vi "Service.Create.vi"(7 "Type":T1, 8 "error in (no error)":errorcluster, 10 "Variant":variant, 11 "Section Ptr":T2 format="%.0x") -> (0 "error out":errorcluster, 3 "Parent Ref out":T2 format="%.0x")   [LabVIEW 2019, in "Diagnostics Addon System Explorer.lvlib"]
uses:
  Diagnostics Addon System Explorer.lvlib
  <vilib>/NI VeriStand/Custom Device API/Custom Device Item Ref.ctl
  Addon Shared/Types/Type.ctl
  Types/Frame.Export.ctl
  Addon Shared/Types/Signal.ctl
  Types/FG.Action.ctl
  Types/CmdResp.Export.ctl
  Types/IO.Export.ctl
  Types/Poll.Create.ctl
  Types/Poll.Settings.ctl
  Types/Poll.LinkedNode.ctl
  Addon Shared/Types/DPID.Rate.ctl
  Addon Shared/Types/DPID.ctl
  Types/UserDefinedMessage.Export.ctl
  Addon Shared/Types/Security.ctl
  Addon Shared/Types/Security.Type.ctl
  <vilib>/NI VeriStand/Custom Device API/Custom Device Channel.ctl
  <vilib>/NI VeriStand/Custom Device API/Custom Device Channel Type.ctl
  Addon Shared/Types/DTC.Settings.ctl
  Addon Shared/Types/DTC.Descriptor.ctl
  FileDependency.Create.vi
  Addon Shared/SubVIs/Constants.vi
  <vilib>/NI/NI VeriStand Advanced SysDef API/SysDef API/SysDef.Property.Set.vi
  <vilib>/NI/NI VeriStand Advanced SysDef API/_SubVIs/SysDef.Property.Set.U32.vi
  <vilib>/NI VeriStand/Custom Device API/NI VeriStand - Get Item Property.vi
  <vilib>/NI VeriStand/Custom Device API/Get Item Property (U32).vi
  <vilib>/NI/NI VeriStand Advanced SysDef API/_SubVIs/SysDef.Property.Set.U32.Array.vi
  <vilib>/NI VeriStand/Custom Device API/Get Item Property (U32 Array).vi
  FileDependency.Get.Target Path.vi
  <vilib>/Utility/MD5Checksum.llb/MD5Checksum File.vi
  <vilib>/NI/NI VeriStand Advanced SysDef API/_SubVIs/SysDef.Property.Set.DependentFile.vi
  <vilib>/NI/NI VeriStand Advanced SysDef API/SysDef API/SysDef.Property.Remove.vi
  <vilib>/NI/NI VeriStand Advanced SysDef API/_SubVIs/SysDef.Property.Set.I32.vi
  <vilib>/NI/NI VeriStand Advanced SysDef API/_SubVIs/SysDef.Property.Set.DBL.Array.vi
  <vilib>/NI/NI VeriStand Advanced SysDef API/_SubVIs/SysDef.Property.Set.String.Array.vi
  <vilib>/NI VeriStand/Custom Device API/Get Item Property (I32).vi
  <vilib>/NI VeriStand/Custom Device API/Get Item Property (Double Array).vi
  <vilib>/NI VeriStand/Custom Device API/Get Item Property (String Array).vi
  Addon Shared/Diagnostics Addon Shared.lvlib
  <vilib>/NI/NI VeriStand Advanced SysDef API/SysDef API/Advanced System Definition.lvlib
  <vilib>/NI VeriStand/Custom Device API/Custom Device API.lvlib
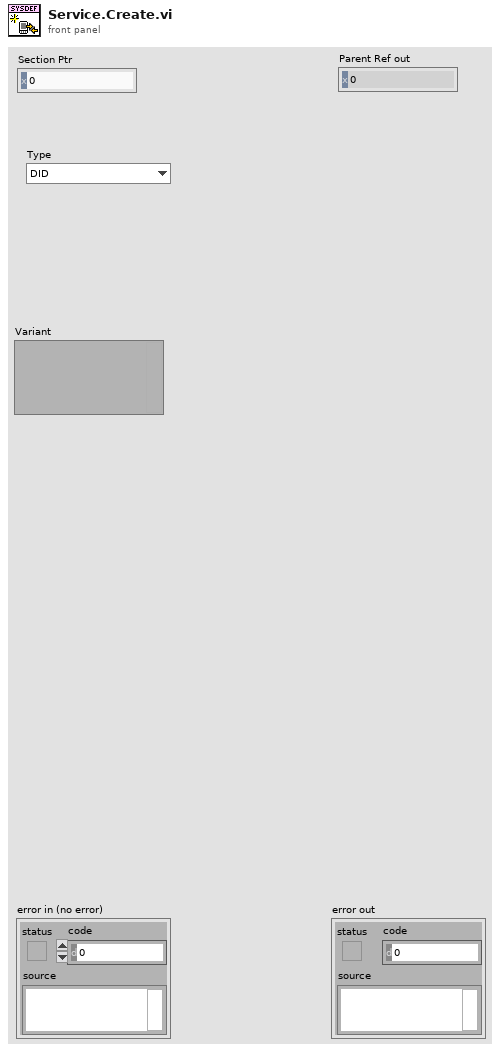
[diagram p1: front panel]
types:
  T1 = typedef "Diagnostics Addon Shared.lvlib/Type.ctl" = enum16{"DID", "CDID", "PID", "CPID", "Read Memory", "Write Memory", "IO Control", "Routine Start", "Routine Request", "Routine Stop", "User Defined", "DTC Control", "Clear DTCs", "Read DTCs", "Start DTCs", "DTC Change Count", "Tester Present", "Unlock ECU", "Reset ECU", "Diag Session Control", "Communication Control", "DPID Control", "Poll Control", "Diag CAN Control"}
  T2 = typedef "Custom Device API.lvlib/Custom Device Item Ref.ctl" = u64
  T3 = typedef "Diagnostics Addon System Explorer.lvlib/Frame.Export.ctl" = cluster{"Name":string, "ID":u32, "Signals":T4[]}
  T4 = typedef "Diagnostics Addon Shared.lvlib/Signal.ctl" = cluster{"Start Bit":u32, "Length":u32, "Scaling Factor":dbl, "Scaling Offset":dbl, "Minimum":dbl, "Maximum":dbl, "Data Type":u32, "Byte Order":u32, "Default Value":dbl, "Name":string, "Units":string}
  T5 = typedef "Diagnostics Addon System Explorer.lvlib/FG.Action.ctl" = enum16{"Get", "Set"}
  T6 = typedef "Diagnostics Addon System Explorer.lvlib/CmdResp.Export.ctl" = cluster{"Cmd":T4[], "Response":T4[]}
  T7 = typedef "Diagnostics Addon System Explorer.lvlib/IO.Export.ctl" = cluster{"Name":string, "ID":u16, "Signals":T6}
  T8 = typedef "Diagnostics Addon System Explorer.lvlib/Poll.Create.ctl" = cluster{"Name":string, "Settings":T9}
  T9 = typedef "Diagnostics Addon System Explorer.lvlib/Poll.Settings.ctl" = cluster{"Input Channels":T10[], "Speed":T11}
  T10 = typedef "Diagnostics Addon System Explorer.lvlib/Poll.LinkedNode.ctl" = cluster{"Node ID":u64}
  T11 = typedef "Diagnostics Addon Shared.lvlib/DPID.Rate.ctl" = enum16{"Slow", "Medium", "Fast"}
  T12 = typedef "Diagnostics Addon Shared.lvlib/DPID.ctl" = cluster{"DPID ID":u8, "Speed":T11, "PIDs":u16[]}
  T13 = typedef "Diagnostics Addon System Explorer.lvlib/UserDefinedMessage.Export.ctl" = cluster{"Name":string, "Signals":T6}
  T14 = typedef "Diagnostics Addon Shared.lvlib/Security.ctl" = cluster{"Type":T15, "Source DLL Path":path, "Target DLL Path":path, "Security Level":u8}
  T15 = typedef "Diagnostics Addon Shared.lvlib/Security.Type.ctl" = enum16{"None", "DLL", "MasterKey"}
  T16 = typedef "Custom Device API.lvlib/Custom Device Channel.ctl" = cluster{"Type":T17, "Units":string, "Default Value":dbl, "Faultable":bool, "Scalable":bool}
  T17 = typedef "Custom Device API.lvlib/Custom Device Channel Type.ctl" = enum16{"Input", "Output"}
  T18 = typedef "Diagnostics Addon Shared.lvlib/DTC.Settings.ctl" = cluster{"Descriptor":T19, "Value.Code":dbl[], "Value.String":string[], "Value.J2012String":string[], "Status.Code":dbl[], "Status.String":string[]}
  T19 = typedef "Diagnostics Addon Shared.lvlib/DTC.Descriptor.ctl" = cluster{"DTC Byte Length":i32, "Status Byte Length":i32, "Add Data Byte Length":i32, "Byte Order":enum16{"Motorola", "Intel"}}
  T20 = typedef "Diagnostics Addon Shared.lvlib/Protocol.ctl" = enum16{"GMLAN", "KWP-2000", "UDS", "User-Defined"}
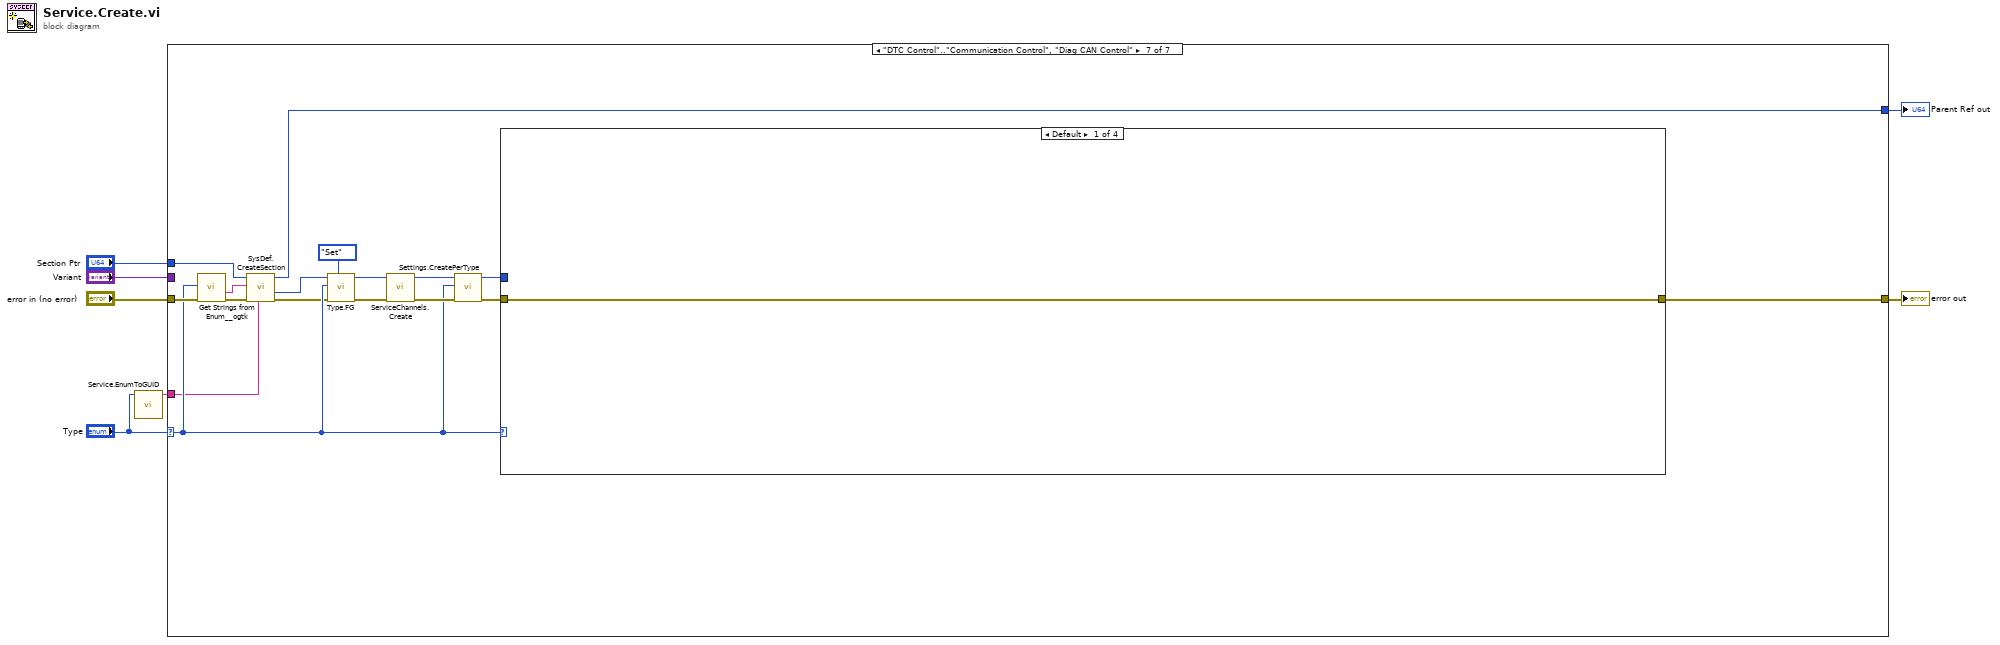
[diagram p0: block diagram]
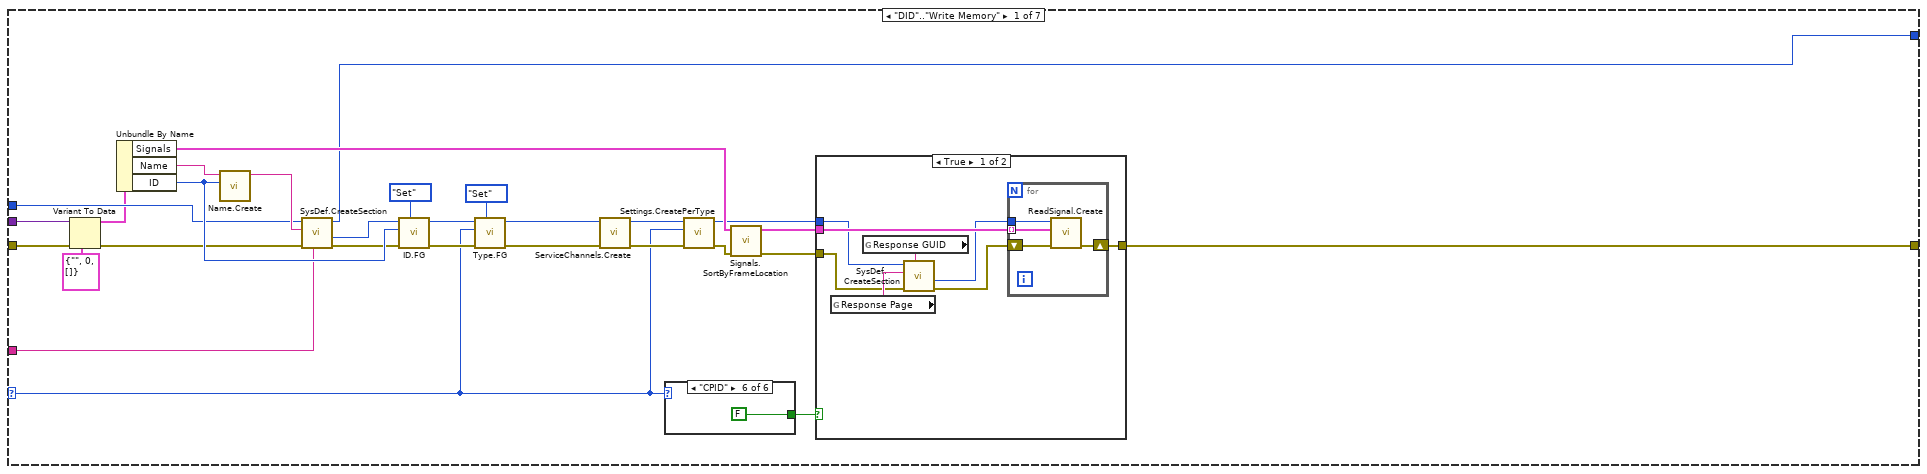
[diagram p2: hidden frame]
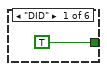
[diagram p3: hidden frame]
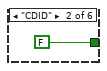
[diagram p4: hidden frame]
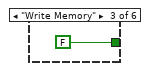
[diagram p5: hidden frame]
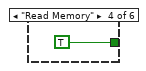
[diagram p6: hidden frame]
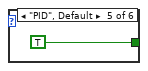
[diagram p7: hidden frame]
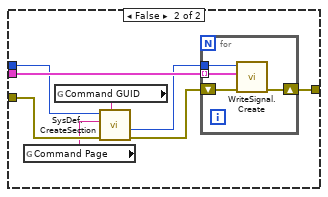
[diagram p8: hidden frame]
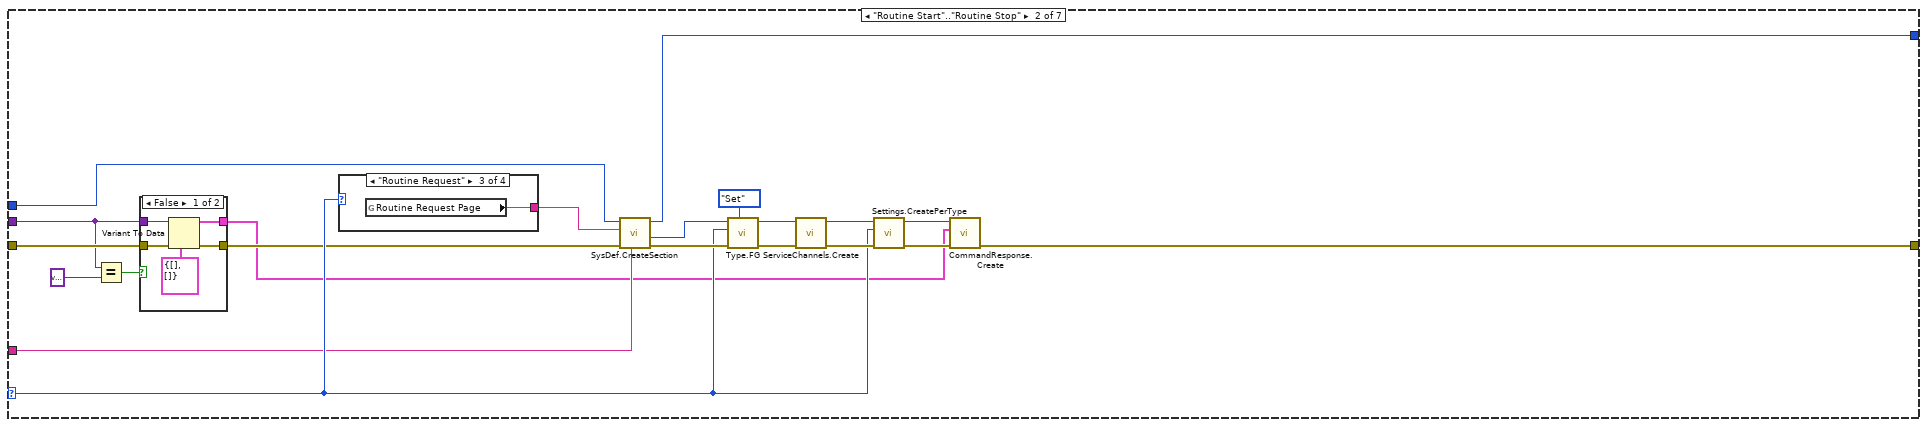
[diagram p9: hidden frame]
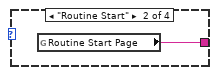
[diagram p12: hidden frame]
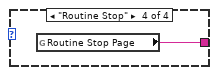
[diagram p13: hidden frame]
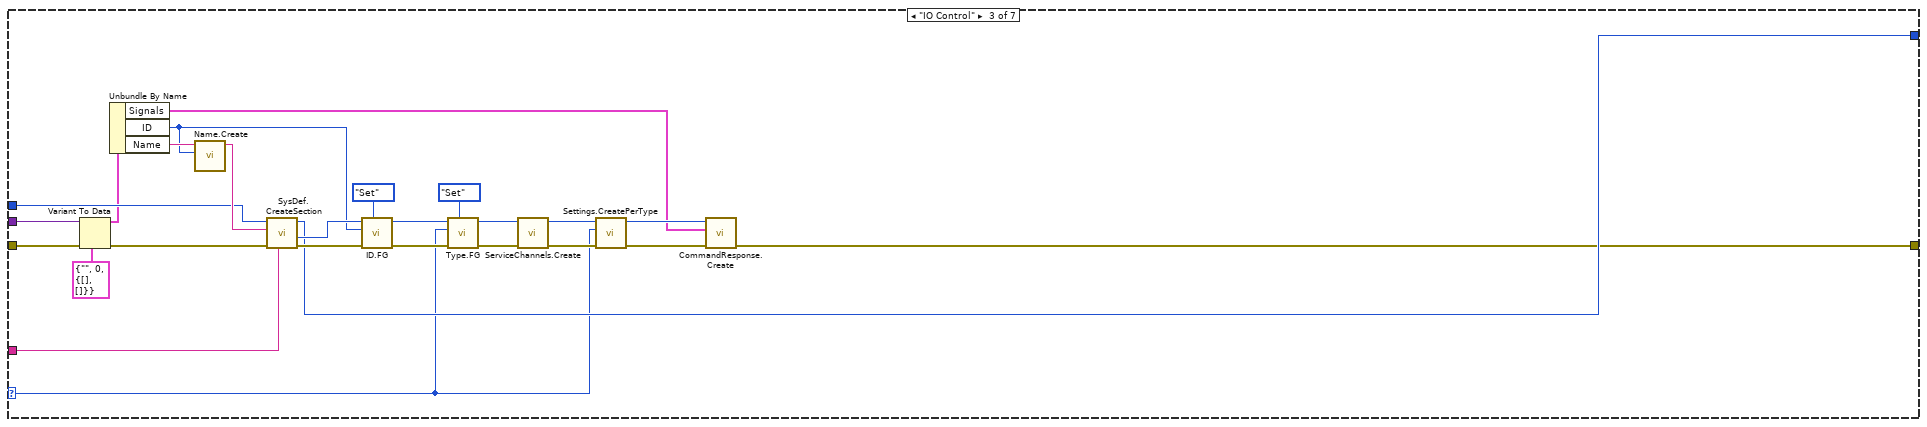
[diagram p14: hidden frame]
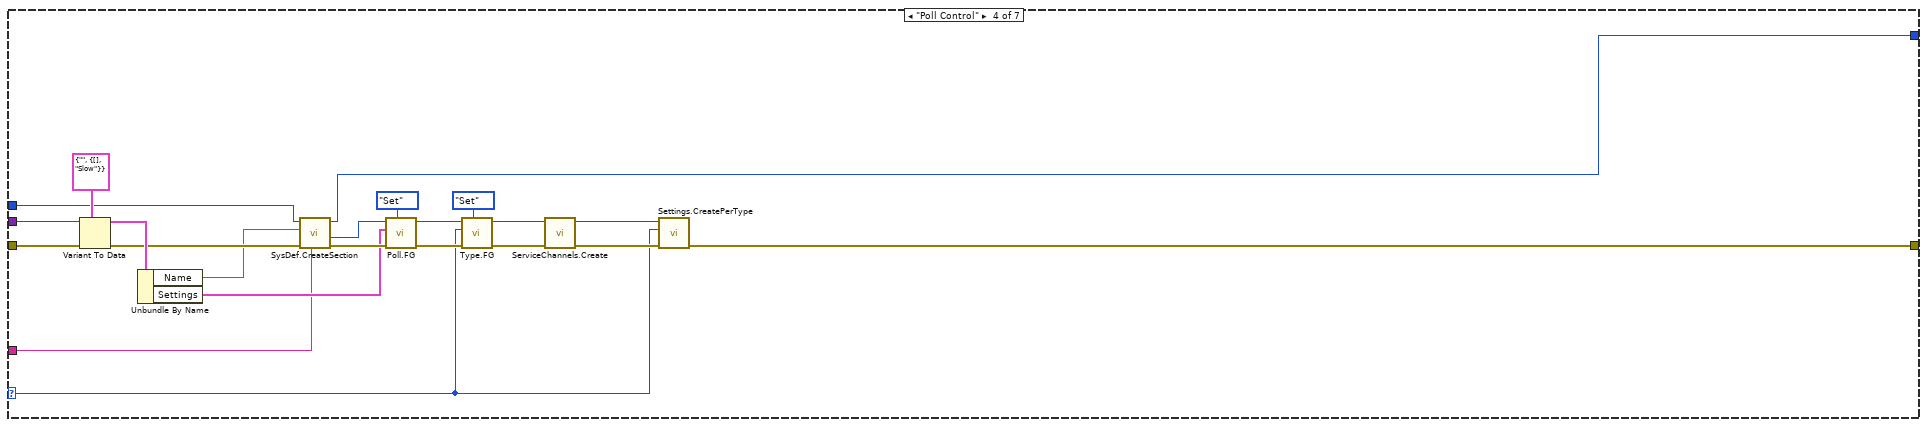
[diagram p15: hidden frame]
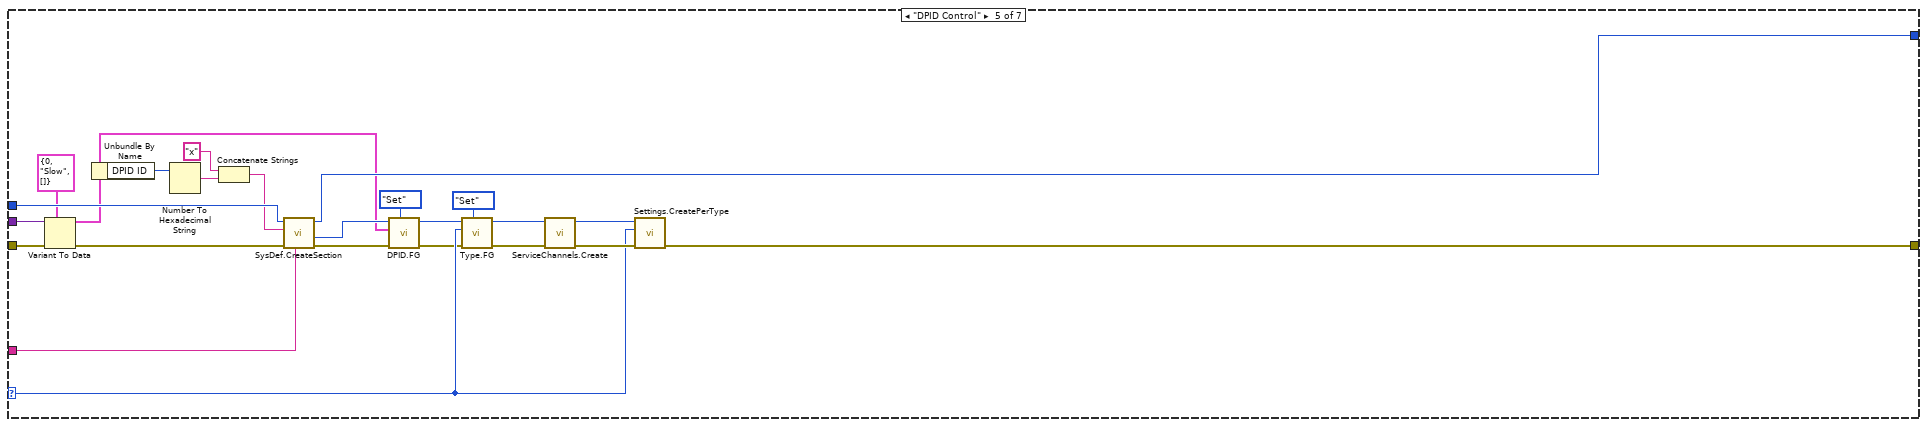
[diagram p16: hidden frame]
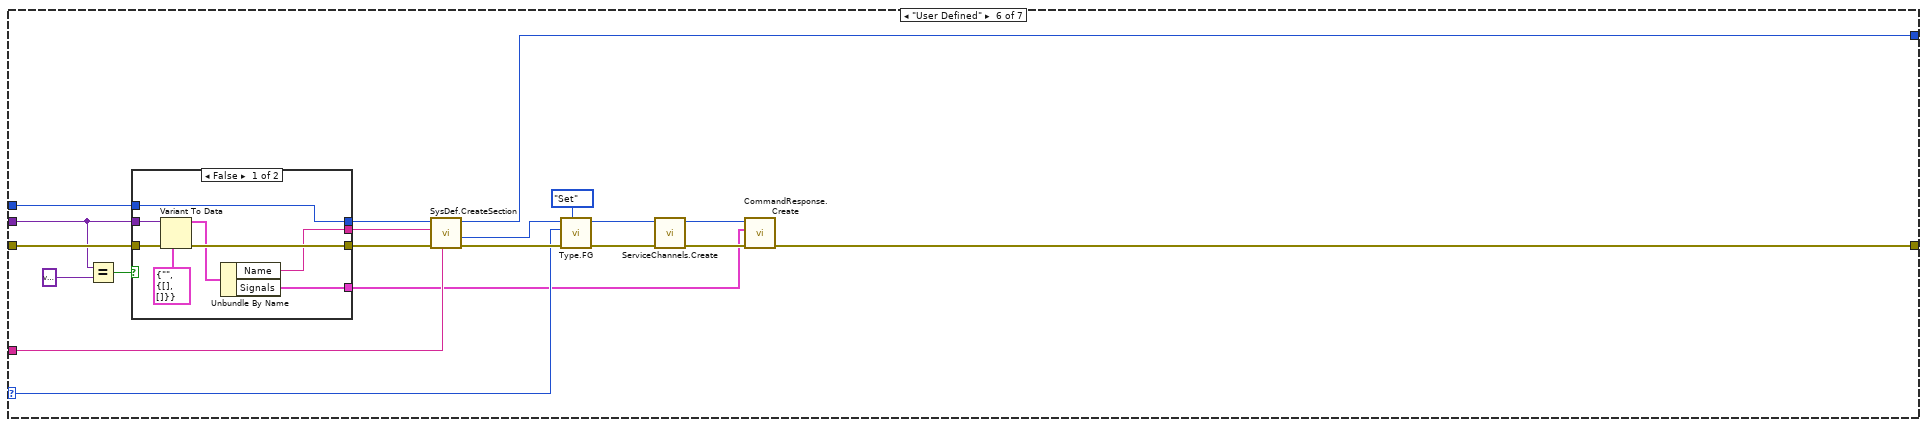
[diagram p17: hidden frame]
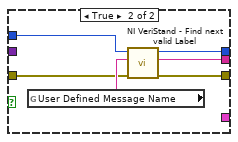
[diagram p18: hidden frame]
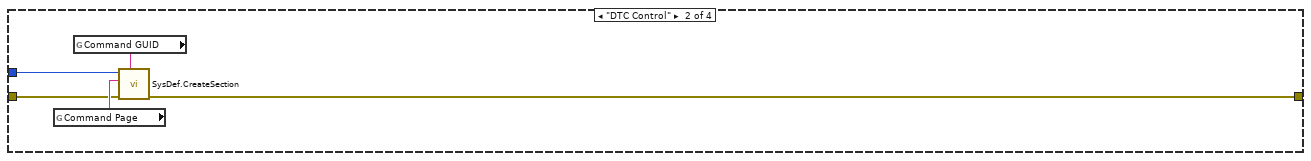
[diagram p19: hidden frame]
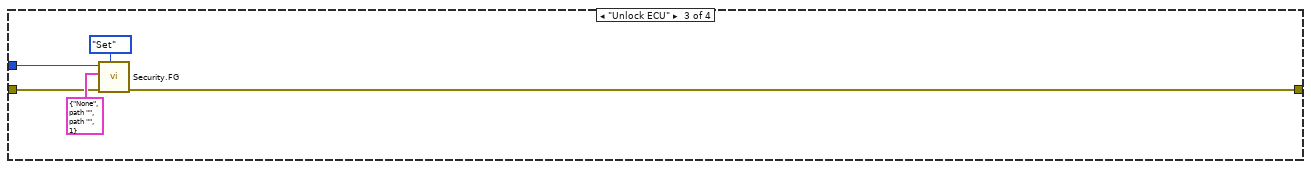
[diagram p20: hidden frame]
diagram:
  n1 = call "Service.EnumToGUID.vi"("Type"="Type") -> ("GUID"=w1:string)  [unwired: 10 in]
  n2 = case shown="\"DTC Control\"..\"Communication Control\", \"Diag CAN Control\"" "Type" {
    selector: "Type" -> [w17 w75 w101 w123 w156 w179 w212]
    tunnel: "error in (no error)" -> [w19 w72 w112 w144 w168 w175 w215]
    tunnel: "Section Ptr" -> [w18 w67 w116 w136 w165 w172 w208]
    tunnel: [w16 w87 w114 w124 w157 w188 w211] -> w5
    tunnel: [w15 w85 w115 w135 w164 w187 w210] -> w4
    tunnel: "Variant" -> [w13 w70 w111 w143 w167 w174 _]
    tunnel: w1 -> [w10 w74 w98 w132 w163 w178 w203]
    frame "DID".."Write Memory" {
      n3 = Variant To Data(error in=w19, type=T3 {"Name"="", "ID"=0, "Signals"=[]} ("Frame"), Variant=w13) -> (data=w11:T3, error out=w14:errorcluster)
      n4 = Unbundle By Name(w11) -> ("Signals"=w25:T4[], "Name"=w32:string, "ID"=w34:u32)
      n5 = call "Name.Create.vi"("PID Number"=w34, "PID Name"=w32) -> ("VS Name"=w36:string)  [unwired: 9 in]
      n6 = call <vilib>:"SysDef.CreateSection.vi"("GUID"=w10, "error in (no error)"=w14, "Name"=w36, "nodeID"=w18) -> ("error out"=w29:errorcluster, "New NodeID"=w30:u64, "nodeID out"=w15:u64)  [unwired: 4 in, 1 out]
      n7 = call "ID.FG.vi"("Action"=FG.Action."Set", "error in (no error)"=w29, "ID"=w34, "Device Item Ref in"=w30) -> ("error out"=w28:errorcluster, "Device Item Ref out"=w27:T2)  [unwired: 5 in, 1 out]
      n8 = call "Type.FG.vi"("Action"=FG.Action."Set", "error in (no error)"=w28, "Type"=w17, "Device Item Ref in"=w27) -> ("error out"=w9:errorcluster, "Device Item Ref out"=w8:T2)  [unwired: 5 in, 1 out]
      n9 = call "ServiceChannels.Create.vi"("error in (no error)"=w9, "nodeID in"=w8) -> ("error out"=w20:errorcluster, "nodeID out"=w22:u64)  [unwired: 8 in]
      n10 = case shown="\"CPID\"" w17 {
        tunnel: [TRUE FALSE FALSE TRUE TRUE FALSE] -> w31
        frame "DID" {
        }
        frame "CDID" {
        }
        frame "Write Memory" {
        }
        frame "Read Memory" {
        }
        frame "PID", Default {
        }
        frame "CPID" {
        }
      }
      n11 = call "Settings.CreatePerType.vi"("error in (no error)"=w20, "Type"=w17, "nodeID in"=w22) -> ("error out"=w21:errorcluster, "nodeID out"=w23:u64)  [unwired: 7 in]
      n12 = call "Signals.SortByFrameLocation.vi"("error in (no error)"=w21, "Signals in"=w25) -> ("error out"=w26:errorcluster, "Signals out"=w24:T4[])  [unwired: 8 in]
      n13 = case shown="True" w31 {
        tunnel: w23 -> [w43 w59]
        tunnel: w24 -> [w50 w62]
        tunnel: [w49 w61] -> w16
        tunnel: w26 -> [w45 w60]
        frame True {
          n14 = global read "Constants.vi" "Response Page"() -> (w47:string)
          n15 = global read "Constants.vi" "Response GUID"() -> (w48:string)
          n16 = call <vilib>:"SysDef.CreateSection.vi"("GUID"=w48, "error in (no error)"=w45, "Name"=w47, "nodeID"=w43) -> ("error out"=w46:errorcluster, "New NodeID"=w44:u64)  [unwired: 4 in, 2 out]
          n17 = for {
            shift-right: [w53] -> w49
            shift-left: w46 -> [w54]
            tunnel: w50 -> [w51] mode=indexing
            tunnel: w44 -> [w52]
            n18 = call "ReadSignal.Create.vi"("error in (no error)"=w54, "Signal Parameters"=w51, "Section Ptr"=w52) -> ("error out"=w53:errorcluster)  [unwired: 7 in, 1 out]
          }
        }
        frame False {
          n19 = global read "Constants.vi" "Command Page"() -> (w55:string)
          n20 = global read "Constants.vi" "Command GUID"() -> (w56:string)
          n21 = call <vilib>:"SysDef.CreateSection.vi"("GUID"=w56, "error in (no error)"=w60, "Name"=w55, "nodeID"=w59) -> ("error out"=w57:errorcluster, "New NodeID"=w58:u64)  [unwired: 4 in, 2 out]
          n22 = for {
            shift-right: [w63] -> w61
            shift-left: w57 -> [w65]
            tunnel: w62 -> [w64] mode=indexing
            tunnel: w58 -> [w66]
            n23 = call "WriteSignal.Create.vi"("error in (no error)"=w65, "Signal Parameters"=w64, "Section Ptr"=w66) -> ("error out"=w63:errorcluster)  [unwired: 7 in, 1 out]
          }
        }
      }
    }
    frame "Routine Start".."Routine Stop" {
      n24 = Equal?(x=w70, y=variant) -> (x = y?=w68:bool)
      n25 = case shown="False" w68 {
        tunnel: [w92 w93] -> w73
        tunnel: w72 -> [w91 w93]
        tunnel: [w89 _] -> w71
        tunnel: w70 -> [w88 _]
        frame False {
          n26 = Variant To Data(error in=w91, type=T6 {"Cmd"=[], "Response"=[]} ("Start Parameters"), Variant=w88) -> (data=w89:T6, error out=w92:errorcluster)
        }
        frame True {
        }
      }
      n27 = case shown="\"Routine Request\"" w75 {
        tunnel: [_ w94 w95 w96] -> w86
        frame Default {
        }
        frame "Routine Start" {
          n28 = global read "Constants.vi" "Routine Start Page"() -> (w94:string)
        }
        frame "Routine Request" {
          n29 = global read "Constants.vi" "Routine Request Page"() -> (w95:string)
        }
        frame "Routine Stop" {
          n30 = global read "Constants.vi" "Routine Stop Page"() -> (w96:string)
        }
      }
      n31 = call <vilib>:"SysDef.CreateSection.vi"("GUID"=w74, "error in (no error)"=w73, "Name"=w86, "nodeID"=w67) -> ("error out"=w78:errorcluster, "New NodeID"=w79:u64, "nodeID out"=w85:u64)  [unwired: 4 in, 1 out]
      n32 = call "Type.FG.vi"("Action"=FG.Action."Set", "error in (no error)"=w78, "Type"=w75, "Device Item Ref in"=w79) -> ("error out"=w77:errorcluster, "Device Item Ref out"=w76:T2)  [unwired: 5 in, 1 out]
      n33 = call "ServiceChannels.Create.vi"("error in (no error)"=w77, "nodeID in"=w76) -> ("error out"=w84:errorcluster, "nodeID out"=w83:u64)  [unwired: 8 in]
      n34 = call "Settings.CreatePerType.vi"("error in (no error)"=w84, "Type"=w75, "nodeID in"=w83) -> ("error out"=w81:errorcluster, "nodeID out"=w80:u64)  [unwired: 7 in]
      n35 = call "CommandResponse.Create.vi"("error in (no error)"=w81, "Signals"=w71, "New NodeID"=w80) -> ("error out"=w87:errorcluster)  [unwired: 8 in]
    }
    frame "IO Control" {
      n36 = Variant To Data(error in=w112, type=T7 {"Name"="", "ID"=0, "Signals"={"Cmd"=[], "Response"=[]}} ("IO Control"), Variant=w111) -> (data=w110:T7, error out=w113:errorcluster)
      n37 = Unbundle By Name(w110) -> ("Signals"=w97:T6, "ID"=w118:u16, "Name"=w121:string)
      n38 = call "Name.Create.vi"("PID Number"=w118, "PID Name"=w121) -> ("VS Name"=w122:string)  [unwired: 9 in]
      n39 = call <vilib>:"SysDef.CreateSection.vi"("GUID"=w98, "error in (no error)"=w113, "Name"=w122, "nodeID"=w116) -> ("error out"=w120:errorcluster, "New NodeID"=w119:u64, "nodeID out"=w115:u64)  [unwired: 4 in, 1 out]
      n40 = call "ID.FG.vi"("Action"=FG.Action."Set", "error in (no error)"=w120, "ID"=w118, "Device Item Ref in"=w119) -> ("error out"=w103:errorcluster, "Device Item Ref out"=w100:T2)  [unwired: 5 in, 1 out]
      n41 = call "Type.FG.vi"("Action"=FG.Action."Set", "error in (no error)"=w103, "Type"=w101, "Device Item Ref in"=w100) -> ("error out"=w102:errorcluster, "Device Item Ref out"=w99:T2)  [unwired: 5 in, 1 out]
      n42 = call "ServiceChannels.Create.vi"("error in (no error)"=w102, "nodeID in"=w99) -> ("error out"=w108:errorcluster, "nodeID out"=w107:u64)  [unwired: 8 in]
      n43 = call "Settings.CreatePerType.vi"("error in (no error)"=w108, "Type"=w101, "nodeID in"=w107) -> ("error out"=w105:errorcluster, "nodeID out"=w106:u64)  [unwired: 7 in]
      n44 = call "CommandResponse.Create.vi"("error in (no error)"=w105, "Signals"=w97, "New NodeID"=w106) -> ("error out"=w114:errorcluster)  [unwired: 8 in]
    }
    frame "Poll Control" {
      n45 = Variant To Data(error in=w144, type=T8 {"Name"="", "Settings"={"Input Channels"=[], "Speed"=enum."Slow"}} ("output cluster"), Variant=w143) -> (data=w141:T8, error out=w137:errorcluster)
      n46 = Unbundle By Name(w141) -> ("Name"=w134:string, "Settings"=w133:T9)
      n47 = call <vilib>:"SysDef.CreateSection.vi"("GUID"=w132, "error in (no error)"=w137, "Name"=w134, "nodeID"=w136) -> ("error out"=w139:errorcluster, "New NodeID"=w138:u64, "nodeID out"=w135:u64)  [unwired: 4 in, 1 out]
      n48 = call "Poll.FG.vi"("Action"=FG.Action."Set", "error in"=w139, "Selected Channels"=w133, "Parent Ref"=w138) -> ("error out"=w130:errorcluster, "Parent Ref Out"=w128:T2)  [unwired: 5 in, 1 out]
      n49 = call "Type.FG.vi"("Action"=FG.Action."Set", "error in (no error)"=w130, "Type"=w123, "Device Item Ref in"=w128) -> ("error out"=w129:errorcluster, "Device Item Ref out"=w127:T2)  [unwired: 5 in, 1 out]
      n50 = call "ServiceChannels.Create.vi"("error in (no error)"=w129, "nodeID in"=w127) -> ("error out"=w126:errorcluster, "nodeID out"=w125:u64)  [unwired: 8 in]
      n51 = call "Settings.CreatePerType.vi"("error in (no error)"=w126, "Type"=w123, "nodeID in"=w125) -> ("error out"=w124:errorcluster)  [unwired: 7 in, 1 out]
    }
    frame "DPID Control" {
      n52 = Variant To Data(error in=w168, type=T12 {"DPID ID"=0, "Speed"=enum."Slow", "PIDs"=[]} ("DPID"), Variant=w167) -> (data=w145:T12, error out=w166:errorcluster)
      n53 = Unbundle By Name(w145) -> ("DPID ID"=w153:u8)
      n54 = Number To Hexadecimal String(2:w153) -> (0:w155:string)  [unwired: 1 in]
      n55 = Concatenate Strings("x" ("string"), w155) -> (w151:string)
      n56 = call <vilib>:"SysDef.CreateSection.vi"("GUID"=w163, "error in (no error)"=w166, "Name"=w151, "nodeID"=w165) -> ("error out"=w149:errorcluster, "New NodeID"=w148:u64, "nodeID out"=w164:u64)  [unwired: 4 in, 1 out]
      n57 = call "DPID.FG.vi"("Action"=FG.Action."Set", "error in (no error)"=w149, "DPID"=w145, "Device Item Ref in"=w148) -> ("error out"=w150:errorcluster, "Device Item Ref out"=w147:T2)  [unwired: 5 in, 1 out]
      n58 = call "Type.FG.vi"("Action"=FG.Action."Set", "error in (no error)"=w150, "Type"=w156, "Device Item Ref in"=w147) -> ("error out"=w161:errorcluster, "Device Item Ref out"=w160:T2)  [unwired: 5 in, 1 out]
      n59 = call "ServiceChannels.Create.vi"("error in (no error)"=w161, "nodeID in"=w160) -> ("error out"=w159:errorcluster, "nodeID out"=w158:u64)  [unwired: 8 in]
      n60 = call "Settings.CreatePerType.vi"("error in (no error)"=w159, "Type"=w156, "nodeID in"=w158) -> ("error out"=w157:errorcluster)  [unwired: 7 in, 1 out]
    }
    frame "User Defined" {
      n61 = Equal?(x=w174, y=variant) -> (x = y?=w176:bool)
      n62 = case shown="False" w176 {
        tunnel: [w196 w199] -> w173
        tunnel: w175 -> [w195 w200]
        tunnel: [w191 w198] -> w171
        tunnel: w174 -> [w193 _]
        tunnel: w172 -> [w190 w201]
        tunnel: [w190 w197] -> w170
        tunnel: [w189 _] -> w169
        frame False {
          n63 = Variant To Data(error in=w195, type=T13 {"Name"="", "Signals"={"Cmd"=[], "Response"=[]}} ("IO Control"), Variant=w193) -> (data=w194:T13, error out=w196:errorcluster)
          n64 = Unbundle By Name(w194) -> ("Name"=w191:string, "Signals"=w189:T6)
        }
        frame True {
          n65 = global read "Constants.vi" "User Defined Message Name"() -> (w202:string)
          n66 = call <vilib>:"NI VeriStand - Find next valid Label.vi"("error in (no error)"=w200, "Label"=w202, "Item Ref in"=w201) -> ("error out"=w199:errorcluster, "Label out"=w198:string, "Item Ref out"=w197:T2)  [unwired: 4 in, 2 out]
        }
      }
      n67 = call <vilib>:"SysDef.CreateSection.vi"("GUID"=w178, "error in (no error)"=w173, "Name"=w171, "nodeID"=w170) -> ("error out"=w180:errorcluster, "New NodeID"=w181:u64, "nodeID out"=w187:u64)  [unwired: 4 in, 1 out]
      n68 = call "Type.FG.vi"("Action"=FG.Action."Set", "error in (no error)"=w180, "Type"=w179, "Device Item Ref in"=w181) -> ("error out"=w183:errorcluster, "Device Item Ref out"=w182:T2)  [unwired: 5 in, 1 out]
      n69 = call "ServiceChannels.Create.vi"("error in (no error)"=w183, "nodeID in"=w182) -> ("error out"=w186:errorcluster, "nodeID out"=w185:u64)  [unwired: 8 in]
      n70 = call "CommandResponse.Create.vi"("error in (no error)"=w186, "Signals"=w169, "New NodeID"=w185) -> ("error out"=w188:errorcluster)  [unwired: 8 in]
    }
    frame "DTC Control".."Communication Control", "Diag CAN Control" {
      n71 = call <userlib>:"Get Strings from Enum__ogtk.vi"("error in (no error)"=w215, "Enum"=w212) -> ("error out"=w209:errorcluster, "String Value"=w214:string)  [unwired: 6 in, 2 out]
      n72 = call <vilib>:"SysDef.CreateSection.vi"("GUID"=w203, "error in (no error)"=w209, "Name"=w214, "nodeID"=w208) -> ("error out"=w207:errorcluster, "New NodeID"=w206:u64, "nodeID out"=w210:u64)  [unwired: 4 in, 1 out]
      n73 = call "Type.FG.vi"("Action"=FG.Action."Set", "error in (no error)"=w207, "Type"=w212, "Device Item Ref in"=w206) -> ("error out"=w205:errorcluster, "Device Item Ref out"=w204:T2)  [unwired: 5 in, 1 out]
      n74 = call "ServiceChannels.Create.vi"("error in (no error)"=w205, "nodeID in"=w204) -> ("error out"=w218:errorcluster, "nodeID out"=w219:u64)  [unwired: 8 in]
      n75 = call "Settings.CreatePerType.vi"("error in (no error)"=w218, "Type"=w212, "nodeID in"=w219) -> ("error out"=w217:errorcluster, "nodeID out"=w216:u64)  [unwired: 7 in]
      n76 = case shown="Default" w212 {
        tunnel: [w220 w222 w226 w253] -> w211
        tunnel: w216 -> [_ w223 w227 w251]
        tunnel: w217 -> [w220 w221 w228 w252]
        frame Default {
        }
        frame "DTC Control" {
          n77 = global read "Constants.vi" "Command Page"() -> (w225:string)
          n78 = global read "Constants.vi" "Command GUID"() -> (w224:string)
          n79 = call <vilib>:"SysDef.CreateSection.vi"("GUID"=w224, "error in (no error)"=w221, "Name"=w225, "nodeID"=w223) -> ("error out"=w222:errorcluster)  [unwired: 4 in, 3 out]
        }
        frame "Unlock ECU" {
          n80 = call "Security.FG.vi"("Action"=FG.Action."Set", "error in (no error)"=w228, "Security"=T14 {"Type"=enum."None", "Source DLL Path"=path "", "Target DLL Path"=path "", "Security Level"=1}, "Device Item Ref in"=w227) -> ("error out"=w226:errorcluster)  [unwired: 5 in, 2 out]
        }
        frame "Read DTCs", "Start DTCs" {
          n81 = call "CAN.Protocol.Find.vi"("error in (no error)"=w252, "Node Ptr"=w251) -> ("error out"=w245:errorcluster, "Diagnostic Protocol"=w250:T20, "Section Ref out"=w246:T2)  [unwired: 7 in]
          n82 = case shown="\"User-Defined\"" w250 {
            tunnel: [u32 2 ("Mode ID") u32 3 ("Mode ID") w261 u32 2 ("Mode ID")] -> w244
            tunnel: [u32 1 ("Mode ID") u32 1 ("Mode ID") w261 u32 1 ("Mode ID")] -> w243
            tunnel: [u32 0 ("Mode ID") u32 0 ("Mode ID") w261 u32 0 ("Mode ID")] -> w242
            frame "GMLAN" {
            }
            frame "UDS" {
            }
            frame "User-Defined" {
              w261 = u8 0 ("Mode ID")
            }
            frame "KWP-2000" {
            }
          }
          n83 = Bundle By Name(cluster=T18 {"Descriptor"={"DTC Byte Length"=2, "Status Byte Length"=1, "Add Data Byte Length"=1, "Byte Order"=enum."Motorola"}, "Value.Code"=[], "Value.String"=[], "Value.J2012String"=[], "Status.Code"=[], "Status.String"=[]} ("DTC"), "Descriptor.DTC Byte Length"=w244, "Descriptor.Status Byte Length"=w243, "Descriptor.Add Data Byte Length"=w242) -> (w247:T18)
          n84 = call "DTCDescriptor.FG.vi"("Action"=FG.Action."Set", "error in (no error)"=w245, "DTC"=w247, "Device Item Ref in"=w246) -> ("error out"=w240:errorcluster, "Device Item Ref out"=w239:T2)  [unwired: 5 in, 1 out]
          n85 = global read "Constants.vi" "Response Page"() -> (w238:string)
          n86 = global read "Constants.vi" "Service Response GUID"() -> (w241:string)
          n87 = call <vilib>:"SysDef.CreateSection.vi"("GUID"=w241, "error in (no error)"=w240, "Name"=w238, "nodeID"=w239) -> ("error out"=w234:errorcluster, "New NodeID"=w231:u64)  [unwired: 4 in, 2 out]
          n88 = global read "Constants.vi" "DTCs_# of DTCs"() -> (w236:string)
          n89 = global read "Constants.vi" "Protected Signal GUID"() -> (w235:string)
          n90 = call <vilib>:"SysDef.CreateChannel.vi"("GUID"=w235, "error in (no error)"=w234, "Channel"=T16 {"Type"=enum."Output", "Units"="", "Default Value"=0.0, "Faultable"=FALSE, "Scalable"=FALSE}, "Name"=w236, "nodeID"=w231) -> ("error out"=w233:errorcluster, "nodeID out"=w232:u64)  [unwired: 3 in, 2 out]
          n91 = for {
            N: u32 10 ("t") -> [_]
            tunnel: w232 -> [w272]
            shift-right: [w276] -> w253
            shift-left: w233 -> [w271]
            i -> [w275]
            n92 = global read "Constants.vi" "DTC_Signal Suffix"() -> (w269:string[])
            n93 = global read "Constants.vi" "DTC_Signal Prefix"() -> (w268:string)
            n94 = Increment(x=w275) -> (x+1=w274:i32)
            n95 = Number To Decimal String(number=w274) -> (decimal integer string=w273:string)  [unwired: 1 in]
            n96 = Concatenate Strings(w268, w273) -> (w270:string)
            n97 = global read "Constants.vi" "DTC GUID"() -> (w267:string)
            n98 = call <vilib>:"SysDef.CreateSection.vi"("GUID"=w267, "error in (no error)"=w271, "Name"=w270, "nodeID"=w272) -> ("error out"=w266:errorcluster, "New NodeID"=w265:u64)  [unwired: 4 in, 2 out]
            n99 = for {
              tunnel: w265 -> [w282]
              tunnel: w270 -> [w279]
              tunnel: w269 -> [w280] mode=indexing
              shift-right: [w284] -> w276
              shift-left: w266 -> [w281]
              n100 = global read "Constants.vi" "Protected Signal GUID"() -> (w277:string)
              n101 = Concatenate Strings(w279, w280) -> (w278:string)
              n102 = call <vilib>:"SysDef.CreateChannel.vi"("GUID"=w277, "error in (no error)"=w281, "Channel"=T16 {"Type"=enum."Output", "Units"="", "Default Value"=0.0, "Faultable"=FALSE, "Scalable"=FALSE}, "Name"=w278, "nodeID"=w282) -> ("error out"=w284:errorcluster)  [unwired: 3 in, 3 out]
            }
          }
        }
      }
    }
  }
  "error out" <- w5
  "Parent Ref out" <- w4
